vi "test TCX read (installed 71).vi"() -> ()   [LabVIEW 2011] (continued)
><Trackpoint><Time>2008-03-03T14:08:26Z</Time><Position><LatitudeDegrees>35.866312</LatitudeDegrees><LongitudeDegrees>-78.880611</LongitudeDegrees></Position><AltitudeMeters>99.153</AltitudeMeters><DistanceMeters>10693.477</DistanceMeters><Cadence>84</Cadence><Extensions><TPX xmlns=\"http://www.garmin.com/xmlschemas/ActivityExtension/v2\"><Watts>141</Watts></TPX></Extensions></Trackpoint><Trackpoint><Time>2008-03-03T14:08:27Z</Time><Position><LatitudeDegrees>35.866343</LatitudeDegrees><LongitudeDegrees>-78.880503</LongitudeDegrees></Position><AltitudeMeters>99.153</AltitudeMeters><DistanceMeters>10703.830</DistanceMeters><Cadence>84</Cadence><Extensions><TPX xmlns=\"http://www.garmin.com/xmlschemas/ActivityExtension/v2\"><Watts>141</Watts></TPX></Extensions></Trackpoint><Trackpoint><Time>2008-03-03T14:08:28Z</Time><Position><LatitudeDegrees>35.866345</LatitudeDegrees><LongitudeDegrees>-78.880391</LongitudeDegrees></Position><AltitudeMeters>99.153</AltitudeMeters><DistanceMeters>10713.883</DistanceMeters><Cadence>38</Cadence><Extensions><TPX xmlns=\"http://www.garmin.com/xmlschemas/ActivityExtension/v2\"><Watts>13</Watts></TPX></Extensions></Trackpoint><Trackpoint><Time>2008-03-03T14:08:29Z</Time><Position><LatitudeDegrees>35.866328</LatitudeDegrees><LongitudeDegrees>-78.880294</LongitudeDegrees></Position><AltitudeMeters>99.634</AltitudeMeters><DistanceMeters>10722.747</DistanceMeters><Cadence>36</Cadence><Extensions><TPX xmlns=\"http://www.garmin.com/xmlschemas/ActivityExtension/v2\"><Watts>26</Watts></TPX></Extensions></Trackpoint><Trackpoint><Time>2008-03-03T14:08:30Z</Time><Position><LatitudeDegrees>35.866278</LatitudeDegrees><LongitudeDegrees>-78.880221</LongitudeDegrees></Position><AltitudeMeters>99.634</AltitudeMeters><DistanceMeters>10730.963</DistanceMeters><Cadence>36</Cadence><Extensions><TPX xmlns=\"http://www.garmin.com/xmlschemas/ActivityExtension/v2\"><Watts>25</Watts></TPX></Extensions></Trackpoint><Trackpoint><Time>2008-03-03T14:08:31Z</Time><Position><LatitudeDegrees>35.866190</LatitudeDegrees><LongitudeDegrees>-78.880183</LongitudeDegrees></Position><AltitudeMeters>99.634</AltitudeMeters><DistanceMeters>10741.313</DistanceMeters><Cadence>74</Cadence><Extensions><TPX xmlns=\"http://www.garmin.com/xmlschemas/ActivityExtension/v2\"><Watts>115</Watts></TPX></Extensions></Trackpoint><Trackpoint><Time>2008-03-03T14:08:32Z</Time><Position><LatitudeDegrees>35.866105</LatitudeDegrees><LongitudeDegrees>-78.880147</LongitudeDegrees></Position><AltitudeMeters>99.634</AltitudeMeters><DistanceMeters>10751.273</DistanceMeters><Cadence>74</Cadence><Extensions><TPX xmlns=\"http://www.garmin.com/xmlschemas/ActivityExtension/v2\"><Watts>166</Watts></TPX></Extensions></Trackpoint><Trackpoint><Time>2008-03-03T14:08:33Z</Time><Position><LatitudeDegrees>35.866021</LatitudeDegrees><LongitudeDegrees>-78.880110</LongitudeDegrees></Position><AltitudeMeters>100.115</AltitudeMeters><DistanceMeters>10761.154</DistanceMeters><Cadence>75</Cadence><Extensions><TPX xmlns=\"http://www.garmin.com/xmlschemas/ActivityExtension/v2\"><Watts>323</Watts></TPX></Extensions></Trackpoint><Trackpoint><Time>2008-03-03T14:08:34Z</Time><Position><LatitudeDegrees>35.865940</LatitudeDegrees><LongitudeDegrees>-78.880073</LongitudeDegrees></Position><AltitudeMeters>99.634</AltitudeMeters><DistanceMeters>10770.754</DistanceMeters><Cadence>76</Cadence><Extensions><TPX xmlns=\"http://www.garmin.com/xmlschemas/ActivityExtension/v2\"><Watts>355</Watts></TPX></Extensions></Trackpoint><Trackpoint><Time>2008-03-03T14:08:35Z</Time><Position><LatitudeDegrees>35.865853</LatitudeDegrees><LongitudeDegrees>-78.880034</LongitudeDegrees></Position><AltitudeMeters>100.115</AltitudeMeters><DistanceMeters>10781.071</DistanceMeters><Cadence>77</Cadence><Extensions><TPX xmlns=\"http://www.garmin.com/xmlschemas/ActivityExtension/v2\"><Watts>333</Watts></TPX></Extensions></Trackpoint><Trackpoint><Time>2008-03-03T14:08:36Z</Time><Position><LatitudeDegrees>35.865737</LatitudeDegrees><LongitudeDegrees>-78.879989</LongitudeDegrees></Position><AltitudeMeters>99.153</AltitudeMeters><DistanceMeters>10794.555</DistanceMeters><Cadence>80</Cadence><Extensions><TPX xmlns=\"http://www.garmin.com/xmlschemas/ActivityExtension/v2\"><Watts>223</Watts></TPX></Extensions></Trackpoint><Trackpoint><Time>2008-03-03T14:08:37Z</Time><Position><LatitudeDegrees>35.865638</LatitudeDegrees><LongitudeDegrees>-78.879966</LongitudeDegrees></Position><AltitudeMeters>99.634</AltitudeMeters><DistanceMeters>10805.750</DistanceMeters><Cadence>80</Cadence><Extensions><TPX xmlns=\"http://www.garmin.com/xmlschemas/ActivityExtension/v2\"><Watts>223</Watts></TPX></Extensions></Trackpoint><Trackpoint><Time>2008-03-03T14:08:38Z</Time><Position><LatitudeDegrees>35.865555</LatitudeDegrees><LongitudeDegrees>-78.879967</LongitudeDegrees></Position><AltitudeMeters>98.672</AltitudeMeters><DistanceMeters>10814.789</DistanceMeters><Cadence>83</Cadence><Extensions><TPX xmlns=\"http://www.garmin.com/xmlschemas/ActivityExtension/v2\"><Watts>157</Watts></TPX></Extensions></Trackpoint><Trackpoint><Time>2008-03-03T14:08:39Z</Time><Position><LatitudeDegrees>35.865453</LatitudeDegrees><LongitudeDegrees>-78.879945</LongitudeDegrees></Position><AltitudeMeters>98.672</AltitudeMeters><DistanceMeters>10826.345</DistanceMeters><Cadence>80</Cadence><Extensions><TPX xmlns=\"http://www.garmin.com/xmlschemas/ActivityExtension/v2\"><Watts>148</Watts></TPX></Extensions></Trackpoint><Trackpoint><Time>2008-03-03T14:08:40Z</Time><Position><LatitudeDegrees>35.865353</LatitudeDegrees><LongitudeDegrees>-78.879923</LongitudeDegrees></Position><AltitudeMeters>98.192</AltitudeMeters><DistanceMeters>10837.629</DistanceMeters><Cadence>80</Cadence><Extensions><TPX xmlns=\"http://www.garmin.com/xmlschemas/ActivityExtension/v2\"><Watts>147</Watts></TPX></Extensions></Trackpoint><Trackpoint><Time>2008-03-03T14:08:41Z</Time><Position><LatitudeDegrees>35.865256</LatitudeDegrees><LongitudeDegrees>-78.879904</LongitudeDegrees></Position><AltitudeMeters>97.711</AltitudeMeters><DistanceMeters>10848.521</DistanceMeters><Cadence>85</Cadence><Extensions><TPX xmlns=\"http://www.garmin.com/xmlschemas/ActivityExtension/v2\"><Watts>133</Watts></TPX></Extensions></Trackpoint><Trackpoint><Time>2008-03-03T14:08:42Z</Time><Position><LatitudeDegrees>35.865159</LatitudeDegrees><LongitudeDegrees>-78.879884</LongitudeDegrees></Position><AltitudeMeters>96.750</AltitudeMeters><DistanceMeters>10859.452</DistanceMeters><Cadence>86</Cadence><Extensions><TPX xmlns=\"http://www.garmin.com/xmlschemas/ActivityExtension/v2\"><Watts>132</Watts></TPX></Extensions></Trackpoint><Trackpoint><Time>2008-03-03T14:08:43Z</Time><Position><LatitudeDegrees>35.865057</LatitudeDegrees><LongitudeDegrees>-78.879859</LongitudeDegrees></Position><AltitudeMeters>96.269</AltitudeMeters><DistanceMeters>10871.032</DistanceMeters><Cadence>88</Cadence><Extensions><TPX xmlns=\"http://www.garmin.com/xmlschemas/ActivityExtension/v2\"><Watts>100</Watts></TPX></Extensions></Trackpoint><Trackpoint><Time>2008-03-03T14:08:44Z</Time><Position><LatitudeDegrees>35.864950</LatitudeDegrees><LongitudeDegrees>-78.879828</LongitudeDegrees></Position><AltitudeMeters>95.788</AltitudeMeters><DistanceMeters>10883.138</DistanceMeters><Cadence>84</Cadence><Extensions><TPX xmlns=\"http://www.garmin.com/xmlschemas/ActivityExtension/v2\"><Watts>105</Watts></TPX></Extensions></Trackpoint><Trackpoint><Time>2008-03-03T14:08:45Z</Time><Position><LatitudeDegrees>35.864843</LatitudeDegrees><LongitudeDegrees>-78.879794</LongitudeDegrees></Position><AltitudeMeters>96.269</AltitudeMeters><DistanceMeters>10895.494</DistanceMeters><Cadence>86</Cadence><Extensions><TPX xmlns=\"http://www.garmin.com/xmlschemas/ActivityExtension/v2\"><Watts>123</Watts></TPX></Extensions></Trackpoint><Trackpoint><Time>2008-03-03T14:08:46Z</Time><Position><LatitudeDegrees>35.864733</LatitudeDegrees><LongitudeDegrees>-78.879755</LongitudeDegrees></Position><AltitudeMeters>95.308</AltitudeMeters><DistanceMeters>10908.254</DistanceMeters><Cadence>88</Cadence><Extensions><TPX xmlns=\"http://www.garmin.com/xmlschemas/ActivityExtension/v2\"><Watts>150</Watts></TPX></Extensions></Trackpoint><Trackpoint><Time>2008-03-03T14:08:47Z</Time><Position><LatitudeDegrees>35.864616</LatitudeDegrees><LongitudeDegrees>-78.879705</LongitudeDegrees></Position><AltitudeMeters>94.827</AltitudeMeters><DistanceMeters>10921.946</DistanceMeters><Cadence>88</Cadence><Extensions><TPX xmlns=\"http://www.garmin.com/xmlschemas/ActivityExtension/v2\"><Watts>151</Watts></TPX></Extensions></Trackpoint><Trackpoint><Time>2008-03-03T14:08:48Z</Time><Position><LatitudeDegrees>35.864512</LatitudeDegrees><LongitudeDegrees>-78.879645</LongitudeDegrees></Position><AltitudeMeters>94.347</AltitudeMeters><DistanceMeters>10934.686</DistanceMeters><Cadence>91</Cadence><Extensions><TPX xmlns=\"http://www.garmin.com/xmlschemas/ActivityExtension/v2\"><Watts>156</Watts></TPX></Extensions></Trackpoint><Trackpoint><Time>2008-03-03T14:08:49Z</Time><Position><LatitudeDegrees>35.864420</LatitudeDegrees><LongitudeDegrees>-78.879574</LongitudeDegrees></Position><AltitudeMeters>94.347</AltitudeMeters><DistanceMeters>10946.729</DistanceMeters><Cadence>91</Cadence><Extensions><TPX xmlns=\"http://www.garmin.com/xmlschemas/ActivityExtension/v2\"><Watts>158</Watts></TPX></Extensions></Trackpoint><Trackpoint><Time>2008-03-03T14:08:50Z</Time><Position><LatitudeDegrees>35.864328</LatitudeDegrees><LongitudeDegrees>-78.879493</LongitudeDegrees></Position><AltitudeMeters>94.347</AltitudeMeters><DistanceMeters>10959.344</DistanceMeters><Cadence>91</Cadence><Extensions><TPX xmlns=\"http://www.garmin.com/xmlschemas/ActivityExtension/v2\"><Watts>129</Watts></TPX></Extensions></Trackpoint><Trackpoint><Time>2008-03-03T14:08:51Z</Time><Position><LatitudeDegrees>35.864240</LatitudeDegrees><LongitudeDegrees>-78.879401</LongitudeDegrees></Position><AltitudeMeters>93.385</AltitudeMeters><DistanceMeters>10972.160</DistanceMeters><Cadence>90</Cadence><Extensions><TPX xmlns=\"http://www.garmin.com/xmlschemas/ActivityExtension/v2\"><Watts>124</Watts></TPX></Extensions></Trackpoint><Trackpoint><Time>2008-03-03T14:08:52Z</Time><Position><LatitudeDegrees>35.864158</LatitudeDegrees><LongitudeDegrees>-78.879305</LongitudeDegrees></Position><AltitudeMeters>92.424</AltitudeMeters><DistanceMeters>10984.663</DistanceMeters><Cadence>90</Cadence><Extensions><TPX xmlns=\"http://www.garmin.com/xmlschemas/ActivityExtension/v2\"><Watts>123</Watts></TPX></Extensions></Trackpoint><Trackpoint><Time>2008-03-03T14:08:53Z</Time><Position><LatitudeDegrees>35.864078</LatitudeDegrees><LongitudeDegrees>-78.879213</LongitudeDegrees></Position><AltitudeMeters>92.424</AltitudeMeters><DistanceMeters>10996.836</DistanceMeters><Cadence>87</Cadence><Extensions><TPX xmlns=\"http://www.garmin.com/xmlschemas/ActivityExtension/v2\"><Watts>124</Watts></TPX></Extensions></Trackpoint><Trackpoint><Time>2008-03-03T14:08:54Z</Time><Position><LatitudeDegrees>35.863996</LatitudeDegrees><LongitudeDegrees>-78.879127</LongitudeDegrees></Position><AltitudeMeters>92.424</AltitudeMeters><DistanceMeters>11008.705</DistanceMeters><Cadence>87</Cadence><Extensions><TPX xmlns=\"http://www.garmin.com/xmlschemas/ActivityExtension/v2\"><Watts>124</Watts></TPX></Extensions></Trackpoint><Trackpoint><Time>2008-03-03T14:08:55Z</Time><Position><LatitudeDegrees>35.863928</LatitudeDegrees><LongitudeDegrees>-78.879033</LongitudeDegrees></Position><AltitudeMeters>92.424</AltitudeMeters><DistanceMeters>11020.062</DistanceMeters><Cadence>0</Cadence></Trackpoint><Trackpoint><Time>2008-03-03T14:08:56Z</Time><Position><LatitudeDegrees>35.863913</LatitudeDegrees><LongitudeDegrees>-78.878926</LongitudeDegrees></Position><AltitudeMeters>91.463</AltitudeMeters><DistanceMeters>11029.886</DistanceMeters><Cadence>0</Cadence></Trackpoint><Trackpoint><Time>2008-03-03T14:08:57Z</Time><Position><LatitudeDegrees>35.863940</LatitudeDegrees><LongitudeDegrees>-78.878817</LongitudeDegrees></Position><AltitudeMeters>90.982</AltitudeMeters><DistanceMeters>11040.122</DistanceMeters><Cadence>14</Cadence><Extensions><TPX xmlns=\"http://www.garmin.com/xmlschemas/ActivityExtension/v2\"><Watts>4</Watts></TPX></Extensions></Trackpoint><Trackpoint><Time>2008-03-03T14:08:58Z</Time><Position><LatitudeDegrees>35.864012</LatitudeDegrees><LongitudeDegrees>-78.878736</LongitudeDegrees></Position><AltitudeMeters>90.982</AltitudeMeters><DistanceMeters>11051.058</DistanceMeters><Cadence>73</Cadence><Extensions><TPX xmlns=\"http://www.garmin.com/xmlschemas/ActivityExtension/v2\"><Watts>88</Watts></TPX></Extensions></Trackpoint><Trackpoint><Time>2008-03-03T14:08:59Z</Time><Position><LatitudeDegrees>35.864082</LatitudeDegrees><LongitudeDegrees>-78.878660</LongitudeDegrees></Position><AltitudeMeters>90.982</AltitudeMeters><DistanceMeters>11061.331</DistanceMeters><Cadence>74</Cadence><Extensions><TPX xmlns=\"http://www.garmin.com/xmlschemas/ActivityExtension/v2\"><Watts>121</Watts></TPX></Extensions></Trackpoint><Trackpoint><Time>2008-03-03T14:09:00Z</Time><Position><LatitudeDegrees>35.864150</LatitudeDegrees><LongitudeDegrees>-78.878573</LongitudeDegrees></Position><AltitudeMeters>90.982</AltitudeMeters><DistanceMeters>11072.221</DistanceMeters><Cadence>75</Cadence><Extensions><TPX xmlns=\"http://www.garmin.com/xmlschemas/ActivityExtension/v2\"><Watts>284</Watts></TPX></Extensions></Trackpoint><Trackpoint><Time>2008-03-03T14:09:01Z</Time><Position><LatitudeDegrees>35.864204</LatitudeDegrees><LongitudeDegrees>-78.878489</LongitudeDegrees></Position><AltitudeMeters>91.463</AltitudeMeters><DistanceMeters>11081.919</DistanceMeters><Cadence>76</Cadence><Extensions><TPX xmlns=\"http://www.garmin.com/xmlschemas/ActivityExtension/v2\"><Watts>444</Watts></TPX></Extensions></Trackpoint><Trackpoint><Time>2008-03-03T14:09:02Z</Time><Position><LatitudeDegrees>35.864256</LatitudeDegrees><LongitudeDegrees>-78.878400</LongitudeDegrees></Position><AltitudeMeters>91.943</AltitudeMeters><DistanceMeters>11091.741</DistanceMeters><Cadence>78</Cadence><Extensions><TPX xmlns=\"http://www.garmin.com/xmlschemas/ActivityExtension/v2\"><Watts>540</Watts></TPX></Extensions></Trackpoint><Trackpoint><Time>2008-03-03T14:09:03Z</Time><Position><LatitudeDegrees>35.864308</LatitudeDegrees><LongitudeDegrees>-78.878311</LongitudeDegrees></Position><AltitudeMeters>91.463</AltitudeMeters><DistanceMeters>11101.723</DistanceMeters><Cadence>79</Cadence><Extensions><TPX xmlns=\"http://www.garmin.com/xmlschemas/ActivityExtension/v2\"><Watts>529</Watts></TPX></Extensions></Trackpoint><Trackpoint><Time>2008-03-03T14:09:04Z</Time><Position><LatitudeDegrees>35.864360</LatitudeDegrees><LongitudeDegrees>-78.878217</LongitudeDegrees></Position><AltitudeMeters>91.943</AltitudeMeters><DistanceMeters>11111.980</DistanceMeters><Cadence>79</Cadence><Extensions><TPX xmlns=\"http://www.garmin.com/xmlschemas/ActivityExtension/v2\"><Watts>526</Watts></TPX></Extensions></Trackpoint><Trackpoint><Time>2008-03-03T14:09:05Z</Time><Position><LatitudeDegrees>35.864407</LatitudeDegrees><LongitudeDegrees>-78.878122</LongitudeDegrees></Position><AltitudeMeters>91.943</AltitudeMeters><DistanceMeters>11121.941</DistanceMeters><Cadence>79</Cadence><Extensions><TPX xmlns=\"http://www.garmin.com/xmlschemas/ActivityExtension/v2\"><Watts>475</Watts></TPX></Extensions></Trackpoint><Trackpoint><Time>2008-03-03T14:09:06Z</Time><Position><LatitudeDegrees>35.864447</LatitudeDegrees><LongitudeDegrees>-78.878027</LongitudeDegrees></Position><AltitudeMeters>92.424</AltitudeMeters><DistanceMeters>11131.617</DistanceMeters><Cadence>80</Cadence><Extensions><TPX xmlns=\"http://www.garmin.com/xmlschemas/ActivityExtension/v2\"><Watts>446</Watts></TPX></Extensions></Trackpoint><Trackpoint><Time>2008-03-03T14:09:07Z</Time><Position><LatitudeDegrees>35.864487</LatitudeDegrees><LongitudeDegrees>-78.877926</LongitudeDegrees></Position><AltitudeMeters>92.424</AltitudeMeters><DistanceMeters>11141.777</DistanceMeters><Cadence>80</Cadence><Extensions><TPX xmlns=\"http://www.garmin.com/xmlschemas/ActivityExtension/v2\"><Watts>438</Watts></TPX></Extensions></Trackpoint><Trackpoint><Time>2008-03-03T14:09:08Z</Time><Position><LatitudeDegrees>35.864523</LatitudeDegrees><LongitudeDegrees>-78.877825</LongitudeDegrees></Position><AltitudeMeters>92.424</AltitudeMeters><DistanceMeters>11151.760</DistanceMeters><Cadence>82</Cadence><Extensions><TPX xmlns=\"http://www.garmin.com/xmlschemas/ActivityExtension/v2\"><Watts>413</Watts></TPX></Extensions></Trackpoint><Trackpoint><Time>2008-03-03T14:09:09Z</Time><Position><LatitudeDegrees>35.864554</LatitudeDegrees><LongitudeDegrees>-78.877724</LongitudeDegrees></Position><AltitudeMeters>92.424</AltitudeMeters><DistanceMeters>11161.466</DistanceMeters><Cadence>80</Cadence><Extensions><TPX xmlns=\"http://www.garmin.com/xmlschemas/ActivityExtension/v2\"><Watts>336</Watts></TPX></Extensions></Trackpoint><Trackpoint><Time>2008-03-03T14:09:10Z</Time><Position><LatitudeDegrees>35.864575</LatitudeDegrees><LongitudeDegrees>-78.877624</LongitudeDegrees></Position><AltitudeMeters>91.943</AltitudeMeters><DistanceMeters>11170.762</DistanceMeters><Cadence>80</Cadence><Extensions><TPX xmlns=\"http://www.garmin.com/xmlschemas/ActivityExtension/v2\"><Watts>333</Watts></TPX></Extensions></Trackpoint><Trackpoint><Time>2008-03-03T14:09:11Z</Time><Position><LatitudeDegrees>35.864602</LatitudeDegrees><LongitudeDegrees>-78.877526</LongitudeDegrees></Position><AltitudeMeters>91.943</AltitudeMeters><DistanceMeters>11180.042</DistanceMeters><Cadence>0</Cadence></Trackpoint><Trackpoint><Time>2008-03-03T14:09:12Z</Time><Position><LatitudeDegrees>35.864627</LatitudeDegrees><LongitudeDegrees>-78.877434</LongitudeDegrees></Position><AltitudeMeters>91.463</AltitudeMeters><DistanceMeters>11188.773</DistanceMeters><Cadence>0</Cadence></Trackpoint><Trackpoint><Time>2008-03-03T14:09:13Z</Time><Position><LatitudeDegrees>35.864647</LatitudeDegrees><LongitudeDegrees>-78.877351</LongitudeDegrees></Position><AltitudeMeters>91.463</AltitudeMeters><DistanceMeters>11196.600</DistanceMeters><Cadence>0</Cadence></Trackpoint><Trackpoint><Time>2008-03-03T14:09:14Z</Time><Position><LatitudeDegrees>35.864661</LatitudeDegrees><LongitudeDegrees>-78.877279</LongitudeDegrees></Position><AltitudeMeters>90.982</AltitudeMeters><DistanceMeters>11203.146</DistanceMeters><Cadence>0</Cadence></Trackpoint><Trackpoint><Time>2008-03-03T14:09:15Z</Time><Position><LatitudeDegrees>35.864669</LatitudeDegrees><LongitudeDegrees>-78.877219</LongitudeDegrees></Position><AltitudeMeters>90.982</AltitudeMeters><DistanceMeters>11208.569</DistanceMeters><Cadence>0</Cadence></Trackpoint><Trackpoint><Time>2008-03-03T14:09:16Z</Time><Position><LatitudeDegrees>35.864665</LatitudeDegrees><LongitudeDegrees>-78.877171</LongitudeDegrees></Position><AltitudeMeters>90.501</AltitudeMeters><DistanceMeters>11212.869</DistanceMeters><Cadence>0</Cadence></Trackpoint><Trackpoint><Time>2008-03-03T14:09:17Z</Time><Position><LatitudeDegrees>35.864650</LatitudeDegrees><LongitudeDegrees>-78.877146</LongitudeDegrees></Position><AltitudeMeters>90.501</AltitudeMeters><DistanceMeters>11215.633</DistanceMeters><Cadence>0</Cadence></Trackpoint><Trackpoint><Time>2008-03-03T14:09:18Z</Time><Position><LatitudeDegrees>35.864641</LatitudeDegrees><LongitudeDegrees>-78.877137</LongitudeDegrees></Position><AltitudeMeters>90.501</AltitudeMeters><DistanceMeters>11216.748</DistanceMeters><Cadence>0</Cadence></Trackpoint><Trackpoint><Time>2008-03-03T14:09:19Z</Time><Position><LatitudeDegrees>35.864638</LatitudeDegrees><LongitudeDegrees>-78.877137</LongitudeDegrees></Position><AltitudeMeters>90.501</AltitudeMeters><DistanceMeters>11216.885</DistanceMeters><Cadence>0</Cadence></Trackpoint><Trackpoint><Time>2008-03-03T14:09:20Z</Time><Position><LatitudeDegrees>35.864636</LatitudeDegrees><LongitudeDegrees>-78.877141</LongitudeDegrees></Position><AltitudeMeters>90.021</AltitudeMeters><DistanceMeters>11217.296</DistanceMeters></Trackpoint><Trackpoint><Time>2008-03-03T14:09:21Z</Time><Position><LatitudeDegrees>35.864632</LatitudeDegrees><LongitudeDegrees>-78.877145</LongitudeDegrees></Position><AltitudeMeters>90.501</AltitudeMeters><DistanceMeters>11217.786</DistanceMeters></Trackpoint><Trackpoint><Time>2008-03-03T14:09:22Z</Time></Trackpoint><Trackpoint><Time>2008-03-03T14:09:23Z</Time><Position><LatitudeDegrees>35.864631</LatitudeDegrees><LongitudeDegrees>-78.877146</LongitudeDegrees></Position><AltitudeMeters>90.021</AltitudeMeters><DistanceMeters>11217.786</DistanceMeters></Trackpoint><Trackpoint><Time>2008-03-03T23:05:22Z</Time></Trackpoint><Trackpoint><Time>2008-03-03T23:05:23Z</Time><Position><LatitudeDegrees>35.864599</LatitudeDegrees><LongitudeDegrees>-78.877183</LongitudeDegrees></Position><AltitudeMeters>88.579</AltitudeMeters><DistanceMeters>11217.786</DistanceMeters></Trackpoint></Track></Lap><Lap StartTime=\"2008-03-03T23:05:23Z\"><TotalTimeSeconds>1256.30</TotalTimeSeconds><DistanceMeters>11205.165039</DistanceMeters><MaximumSpeed>14.865000</MaximumSpeed><Calories>380</Calories><Intensity>Active</Intensity><Cadence>76</Cadence><TriggerMethod>Manual</TriggerMethod><Track><Trackpoint><Time>2008-03-03T23:05:24Z</Time><Position><LatitudeDegrees>35.864599</LatitudeDegrees><LongitudeDegrees>-78.877182</LongitudeDegrees></Position><AltitudeMeters>65.026</AltitudeMeters><DistanceMeters>11217.828</DistanceMeters></Trackpoint><Trackpoint><Time>2008-03-03T23:05:25Z</Time><Position><LatitudeDegrees>35.864599</LatitudeDegrees><LongitudeDegrees>-78.877182</LongitudeDegrees></Position><AltitudeMeters>65.026</AltitudeMeters><DistanceMeters>11217.846</DistanceMeters></Trackpoint><Trackpoint><Time>2008-03-03T23:05:26Z</Time><Position><LatitudeDegrees>35.864599</LatitudeDegrees><LongitudeDegrees>-78.877181</LongitudeDegrees></Position><AltitudeMeters>65.026</AltitudeMeters><DistanceMeters>11217.897</DistanceMeters></Trackpoint><Trackpoint><Time>2008-03-03T23:05:27Z</Time><Position><LatitudeDegrees>35.864600</LatitudeDegrees><LongitudeDegrees>-78.877183</LongitudeDegrees></Position><AltitudeMeters>65.026</AltitudeMeters><DistanceMeters>11218.080</DistanceMeters></Trackpoint><Trackpoint><Time>2008-03-03T23:05:28Z</Time><Position><LatitudeDegrees>35.864598</LatitudeDegrees><LongitudeDegrees>-78.877196</LongitudeDegrees></Position><AltitudeMeters>65.026</AltitudeMeters><DistanceMeters>11219.385</DistanceMeters></Trackpoint><Trackpoint><Time>2008-03-03T23:05:29Z</Time><Position><LatitudeDegrees>35.864596</LatitudeDegrees><LongitudeDegrees>-78.877215</LongitudeDegrees></Position><AltitudeMeters>65.026</AltitudeMeters><DistanceMeters>11221.062</DistanceMeters></Trackpoint><Trackpoint><Time>2008-03-03T23:05:30Z</Time><Position><LatitudeDegrees>35.864600</LatitudeDegrees><LongitudeDegrees>-78.877227</LongitudeDegrees></Position><AltitudeMeters>65.026</AltitudeMeters><DistanceMeters>11222.095</DistanceMeters></Trackpoint><Trackpoint><Time>2008-03-03T23:05:31Z</Time><Position><LatitudeDegrees>35.864611</LatitudeDegrees><LongitudeDegrees>-78.877234</LongitudeDegrees></Position><AltitudeMeters>65.026</AltitudeMeters><DistanceMeters>11223.448</DistanceMeters><Cadence>2</Cadence><Extensions><TPX xmlns=\"http://www.garmin.com/xmlschemas/ActivityExtension/v2\"><Watts>194</Watts></TPX></Extensions></Trackpoint><Trackpoint><Time>2008-03-03T23:05:32Z</Time><Position><LatitudeDegrees>35.864624</LatitudeDegrees><LongitudeDegrees>-78.877245</LongitudeDegrees></Position><AltitudeMeters>65.026</AltitudeMeters><DistanceMeters>11225.238</DistanceMeters><Cadence>2</Cadence><Extensions><TPX xmlns=\"http://www.garmin.com/xmlschemas/ActivityExtension/v2\"><Watts>193</Watts></TPX></Extensions></Trackpoint><Trackpoint><Time>2008-03-03T23:05:33Z</Time><Position><LatitudeDegrees>35.864635</LatitudeDegrees><LongitudeDegrees>-78.877267</LongitudeDegrees></Position><AltitudeMeters>65.507</AltitudeMeters><DistanceMeters>11227.559</DistanceMeters><Cadence>0</Cadence></Trackpoint><Trackpoint><Time>2008-03-03T23:05:34Z</Time><Position><LatitudeDegrees>35.864638</LatitudeDegrees><LongitudeDegrees>-78.877295</LongitudeDegrees></Position><AltitudeMeters>65.507</AltitudeMeters><DistanceMeters>11230.062</DistanceMeters><Cadence>20</Cadence><Extensions><TPX xmlns=\"http://www.garmin.com/xmlschemas/ActivityExtension/v2\"><Watts>103</Watts></TPX></Extensions></Trackpoint><Trackpoint><Time>2008-03-03T23:05:35Z</Time><Position><LatitudeDegrees>35.864634</LatitudeDegrees><LongitudeDegrees>-78.877330</LongitudeDegrees></Position><AltitudeMeters>65.507</AltitudeMeters><DistanceMeters>11233.309</DistanceMeters><Cadence>44</Cadence><Extensions><TPX xmlns=\"http://www.garmin.com/xmlschemas/ActivityExtension/v2\"><Watts>320</Watts></TPX></Extensions></Trackpoint><Trackpoint><Time>2008-03-03T23:05:36Z</Time><Position><LatitudeDegrees>35.864623</LatitudeDegrees><LongitudeDegrees>-78.877377</LongitudeDegrees></Position><AltitudeMeters>65.507</AltitudeMeters><DistanceMeters>11237.704</DistanceMeters><Cadence>60</Cadence><Extensions><TPX xmlns=\"http://www.garmin.com/xmlschemas/ActivityExtension/v2\"><Watts>420</Watts></TPX></Extensions></Trackpoint><Trackpoint><Time>2008-03-03T23:05:37Z</Time><Position><LatitudeDegrees>35.864609</LatitudeDegrees><LongitudeDegrees>-78.877434</LongitudeDegrees></Position><AltitudeMeters>65.988</AltitudeMeters><DistanceMeters>11243.220</DistanceMeters><Cadence>60</Cadence><Extensions><TPX xmlns=\"http://www.garmin.com/xmlschemas/ActivityExtension/v2\"><Watts>416</Watts></TPX></Extensions></Trackpoint><Trackpoint><Time>2008-03-03T23:05:38Z</Time><Position><LatitudeDegrees>35.864592</LatitudeDegrees><LongitudeDegrees>-78.877503</LongitudeDegrees></Position><AltitudeMeters>65.988</AltitudeMeters><DistanceMeters>11249.730</DistanceMeters><Cadence>81</Cadence><Extensions><TPX xmlns=\"http://www.garmin.com/xmlschemas/ActivityExtension/v2\"><Watts>637</Watts></TPX></Extensions></Trackpoint><Trackpoint><Time>2008-03-03T23:05:39Z</Time><Position><LatitudeDegrees>35.864574</LatitudeDegrees><LongitudeDegrees>-78.877580</LongitudeDegrees></Position><AltitudeMeters>66.468</AltitudeMeters><DistanceMeters>11257.070</DistanceMeters><Cadence>85</Cadence><Extensions><TPX xmlns=\"http://www.garmin.com/xmlschemas/ActivityExtension/v2\"><Watts>651</Watts></TPX></Extensions></Trackpoint><Trackpoint><Time>2008-03-03T23:05:40Z</Time><Position><LatitudeDegrees>35.864553</LatitudeDegrees><LongitudeDegrees>-78.877662</LongitudeDegrees></Position><AltitudeMeters>66.949</AltitudeMeters><DistanceMeters>11264.834</DistanceMeters><Cadence>72</Cadence><Extensions><TPX xmlns=\"http://www.garmin.com/xmlschemas/ActivityExtension/v2\"><Watts>566</Watts></TPX></Extensions></Trackpoint><Trackpoint><Time>2008-03-03T23:05:41Z</Time><Position><LatitudeDegrees>35.864529</LatitudeDegrees><LongitudeDegrees>-78.877747</LongitudeDegrees></Position><AltitudeMeters>66.949</AltitudeMeters><DistanceMeters>11272.925</DistanceMeters><Cadence>75</Cadence><Extensions><TPX xmlns=\"http://www.garmin.com/xmlschemas/ActivityExtension/v2\"><Watts>522</Watts></TPX></Extensions></Trackpoint><Trackpoint><Time>2008-03-03T23:05:42Z</Time><Position><LatitudeDegrees>35.864500</LatitudeDegrees><LongitudeDegrees>-78.877836</LongitudeDegrees></Position><AltitudeMeters>66.949</AltitudeMeters><DistanceMeters>11281.620</DistanceMeters><Cadence>80</Cadence><Extensions><TPX xmlns=\"http://www.garmin.com/xmlschemas/ActivityExtension/v2\"><Watts>518</Watts></TPX></Extensions></Trackpoint><Trackpoint><Time>2008-03-03T23:05:43Z</Time><Position><LatitudeDegrees>35.864469</LatitudeDegrees><LongitudeDegrees>-78.877929</LongitudeDegrees></Position><AltitudeMeters>66.949</AltitudeMeters><DistanceMeters>11290.788</DistanceMeters><Cadence>86</Cadence><Extensions><TPX xmlns=\"http://www.garmin.com/xmlschemas/ActivityExtension/v2\"><Watts>564</Watts></TPX></Extensions></Trackpoint><Trackpoint><Time>2008-03-03T23:05:44Z</Time><Position><LatitudeDegrees>35.864435</LatitudeDegrees><LongitudeDegrees>-78.878027</LongitudeDegrees></Position><AltitudeMeters>66.949</AltitudeMeters><DistanceMeters>11300.357</DistanceMeters><Cadence>88</Cadence><Extensions><TPX xmlns=\"http://www.garmin.com/xmlschemas/ActivityExtension/v2\"><Watts>556</Watts></TPX></Extensions></Trackpoint><Trackpoint><Time>2008-03-03T23:05:45Z</Time><Position><LatitudeDegrees>35.864399</LatitudeDegrees><LongitudeDegrees>-78.878127</LongitudeDegrees></Position><AltitudeMeters>67.430</AltitudeMeters><DistanceMeters>11310.256</DistanceMeters><Cadence>91</Cadence><Extensions><TPX xmlns=\"http://www.garmin.com/xmlschemas/ActivityExtension/v2\"><Watts>521</Watts></TPX></Extensions></Trackpoint><Trackpoint><Time>2008-03-03T23:05:46Z</Time><Position><LatitudeDegrees>35.864360</LatitudeDegrees><LongitudeDegrees>-78.878227</LongitudeDegrees></Position><AltitudeMeters>67.430</AltitudeMeters><DistanceMeters>11320.329</DistanceMeters><Cadence>86</Cadence><Extensions><TPX xmlns=\"http://www.garmin.com/xmlschemas/ActivityExtension/v2\"><Watts>484</Watts></TPX></Extensions></Trackpoint><Trackpoint><Time>2008-03-03T23:05:47Z</Time><Position><LatitudeDegrees>35.864317</LatitudeDegrees><LongitudeDegrees>-78.878326</LongitudeDegrees></Position><AltitudeMeters>67.430</AltitudeMeters><DistanceMeters>11330.483</DistanceMeters><Cadence>86</Cadence><Extensions><TPX xmlns=\"http://www.garmin.com/xmlschemas/ActivityExtension/v2\"><Watts>487</Watts></TPX></Extensions></Trackpoint><Trackpoint><Time>2008-03-03T23:05:48Z</Time><Position><LatitudeDegrees>35.864267</LatitudeDegrees><LongitudeDegrees>-78.878422</LongitudeDegrees></Position><AltitudeMeters>66.949</AltitudeMeters><DistanceMeters>11340.710</DistanceMeters><Cadence>83</Cadence><Extensions><TPX xmlns=\"http://www.garmin.com/xmlschemas/ActivityExtension/v2\"><Watts>282</Watts></TPX></Extensions></Trackpoint><Trackpoint><Time>2008-03-03T23:05:49Z</Time><Position><LatitudeDegrees>35.864211</LatitudeDegrees><LongitudeDegrees>-78.878514</LongitudeDegrees></Position><AltitudeMeters>66.949</AltitudeMeters><DistanceMeters>11351.038</DistanceMeters><Cadence>84</Cadence><Extensions><TPX xmlns=\"http://www.garmin.com/xmlschemas/ActivityExtension/v2\"><Watts>235</Watts></TPX></Extensions></Trackpoint><Trackpoint><Time>2008-03-03T23:05:50Z</Time><Position><LatitudeDegrees>35.864151</LatitudeDegrees><LongitudeDegrees>-78.878601</LongitudeDegrees></Position><AltitudeMeters>66.949</AltitudeMeters><DistanceMeters>11361.405</DistanceMeters><Cadence>84</Cadence><Extensions><TPX xmlns=\"http://www.garmin.com/xmlschemas/ActivityExtension/v2\"><Watts>191</Watts></TPX></Extensions></Trackpoint><Trackpoint><Time>2008-03-03T23:05:51Z</Time><Position><LatitudeDegrees>35.864086</LatitudeDegrees><LongitudeDegrees>-78.878684</LongitudeDegrees></Position><AltitudeMeters>66.949</AltitudeMeters><DistanceMeters>11371.760</DistanceMeters><Cadence>84</Cadence><Extensions><TPX xmlns=\"http://www.garmin.com/xmlschemas/ActivityExtension/v2\"><Watts>191</Watts></TPX></Extensions></Trackpoint><Trackpoint><Time>2008-03-03T23:05:52Z</Time><Position><LatitudeDegrees>35.864017</LatitudeDegrees><LongitudeDegrees>-78.878758</LongitudeDegrees></Position><AltitudeMeters>66.949</AltitudeMeters><DistanceMeters>11381.933</DistanceMeters><Cadence>0</Cadence></Trackpoint><Trackpoint><Time>2008-03-03T23:05:53Z</Time><Position><LatitudeDegrees>35.863958</LatitudeDegrees><LongitudeDegrees>-78.878832</LongitudeDegrees></Position><AltitudeMeters>66.468</AltitudeMeters><DistanceMeters>11391.171</DistanceMeters><Cadence>0</Cadence></Trackpoint><Trackpoint><Time>2008-03-03T23:05:54Z</Time><Position><LatitudeDegrees>35.863937</LatitudeDegrees><LongitudeDegrees>-78.878942</LongitudeDegrees></Position><AltitudeMeters>65.507</AltitudeMeters><DistanceMeters>11401.371</DistanceMeters><Cadence>17</Cadence></Trackpoint><Trackpoint><Time>2008-03-03T23:05:55Z</Time><Position><LatitudeDegrees>35.863962</LatitudeDegrees><LongitudeDegrees>-78.879042</LongitudeDegrees></Position><AltitudeMeters>65.026</AltitudeMeters><DistanceMeters>11410.849</DistanceMeters><Cadence>74</Cadence><Extensions><TPX xmlns=\"http://www.garmin.com/xmlschemas/ActivityExtension/v2\"><Watts>416</Watts></TPX></Extensions></Trackpoint><Trackpoint><Time>2008-03-03T23:05:56Z</Time><Position><LatitudeDegrees>35.864024</LatitudeDegrees><LongitudeDegrees>-78.879109</LongitudeDegrees></Position><AltitudeMeters>65.507</AltitudeMeters><DistanceMeters>11420.108</DistanceMeters><Cadence>77</Cadence><Extensions><TPX xmlns=\"http://www.garmin.com/xmlschemas/ActivityExtension/v2\"><Watts>616</Watts></TPX></Extensions></Trackpoint><Trackpoint><Time>2008-03-03T23:05:57Z</Time><Position><LatitudeDegrees>35.864098</LatitudeDegrees><LongitudeDegrees>-78.879162</LongitudeDegrees></Position><AltitudeMeters>65.507</AltitudeMeters><DistanceMeters>11429.607</DistanceMeters><Cadence>77</Cadence><Extensions><TPX xmlns=\"http://www.garmin.com/xmlschemas/ActivityExtension/v2\"><Watts>628</Watts></TPX></Extensions></Trackpoint><Trackpoint><Time>2008-03-03T23:05:58Z</Time><Position><LatitudeDegrees>35.864171</LatitudeDegrees><LongitudeDegrees>-78.879226</LongitudeDegrees></Position><AltitudeMeters>65.507</AltitudeMeters><DistanceMeters>11439.525</DistanceMeters><Cadence>81</Cadence><Extensions><TPX xmlns=\"http://www.garmin.com/xmlschemas/ActivityExtension/v2\"><Watts>655</Watts></TPX></Extensions></Trackpoint><Trackpoint><Time>2008-03-03T23:05:59Z</Time><Position><LatitudeDegrees>35.864244</LatitudeDegrees><LongitudeDegrees>-78.879299</LongitudeDegrees></Position><AltitudeMeters>65.507</AltitudeMeters><DistanceMeters>11449.930</DistanceMeters><Cadence>81</Cadence><Extensions><TPX xmlns=\"http://www.garmin.com/xmlschemas/ActivityExtension/v2\"><Watts>662</Watts></TPX></Extensions></Trackpoint><Trackpoint><Time>2008-03-03T23:06:00Z</Time><Position><LatitudeDegrees>35.864320</LatitudeDegrees><LongitudeDegrees>-78.879379</LongitudeDegrees></Position><AltitudeMeters>65.988</AltitudeMeters><DistanceMeters>11461.130</DistanceMeters><Cadence>93</Cadence><Extensions><TPX xmlns=\"http://www.garmin.com/xmlschemas/ActivityExtension/v2\"><Watts>898</Watts></TPX></Extensions></Trackpoint><Trackpoint><Time>2008-03-03T23:06:01Z</Time><Position><LatitudeDegrees>35.864401</LatitudeDegrees><LongitudeDegrees>-78.879461</LongitudeDegrees></Position><AltitudeMeters>65.988</AltitudeMeters><DistanceMeters>11472.757</DistanceMeters><Cadence>93</Cadence><Extensions><TPX xmlns=\"http://www.garmin.com/xmlschemas/ActivityExtension/v2\"><Watts>896</Watts></TPX></Extensions></Trackpoint><Trackpoint><Time>2008-03-03T23:06:02Z</Time><Position><LatitudeDegrees>35.864484</LatitudeDegrees><LongitudeDegrees>-78.879540</LongitudeDegrees></Position><AltitudeMeters>65.988</AltitudeMeters><DistanceMeters>11484.492</DistanceMeters><Cadence>95</Cadence><Extensions><TPX xmlns=\"http://www.garmin.com/xmlschemas/ActivityExtension/v2\"><Watts>957</Watts></TPX></Extensions></Trackpoint><Trackpoint><Time>2008-03-03T23:06:03Z</Time><Position><LatitudeDegrees>35.864573</LatitudeDegrees><LongitudeDegrees>-78.879612</LongitudeDegrees></Position><AltitudeMeters>66.949</AltitudeMeters><DistanceMeters>11496.220</DistanceMeters><Cadence>95</Cadence><Extensions><TPX xmlns=\"http://www.garmin.com/xmlschemas/ActivityExtension/v2\"><Watts>921</Watts></TPX></Extensions></Trackpoint><Trackpoint><Time>2008-03-03T23:06:04Z</Time><Position><LatitudeDegrees>35.864665</LatitudeDegrees><LongitudeDegrees>-78.879671</LongitudeDegrees></Position><AltitudeMeters>67.430</AltitudeMeters><DistanceMeters>11507.750</DistanceMeters><Cadence>94</Cadence><Extensions><TPX xmlns=\"http://www.garmin.com/xmlschemas/ActivityExtension/v2\"><Watts>831</Watts></TPX></Extensions></Trackpoint><Trackpoint><Time>2008-03-03T23:06:05Z</Time><Position><LatitudeDegrees>35.864761</LatitudeDegrees><LongitudeDegrees>-78.879719</LongitudeDegrees></Position><AltitudeMeters>68.872</AltitudeMeters><DistanceMeters>11519.301</DistanceMeters><Cadence>94</Cadence><Extensions><TPX xmlns=\"http://www.garmin.com/xmlschemas/ActivityExtension/v2\"><Watts>728</Watts></TPX></Extensions></Trackpoint><Trackpoint><Time>2008-03-03T23:06:06Z</Time><Position><LatitudeDegrees>35.864857</LatitudeDegrees><LongitudeDegrees>-78.879755</LongitudeDegrees></Position><AltitudeMeters>69.352</AltitudeMeters><DistanceMeters>11530.362</DistanceMeters><Cadence>86</Cadence><Extensions><TPX xmlns=\"http://www.garmin.com/xmlschemas/ActivityExtension/v2\"><Watts>484</Watts></TPX></Extensions></Trackpoint><Trackpoint><Time>2008-03-03T23:06:07Z</Time><Position><LatitudeDegrees>35.864948</LatitudeDegrees><LongitudeDegrees>-78.879780</LongitudeDegrees></Position><AltitudeMeters>69.352</AltitudeMeters><DistanceMeters>11540.706</DistanceMeters><Cadence>83</Cadence><Extensions><TPX xmlns=\"http://www.garmin.com/xmlschemas/ActivityExtension/v2\"><Watts>323</Watts></TPX></Extensions></Trackpoint><Trackpoint><Time>2008-03-03T23:06:08Z</Time><Position><LatitudeDegrees>35.865035</LatitudeDegrees><LongitudeDegrees>-78.879798</LongitudeDegrees></Position><AltitudeMeters>69.833</AltitudeMeters><DistanceMeters>11550.413</DistanceMeters><Cadence>79</Cadence><Extensions><TPX xmlns=\"http://www.garmin.com/xmlschemas/ActivityExtension/v2\"><Watts>321</Watts></TPX></Extensions></Trackpoint><Trackpoint><Time>2008-03-03T23:06:09Z</Time><Position><LatitudeDegrees>35.865119</LatitudeDegrees><LongitudeDegrees>-78.879812</LongitudeDegrees></Position><AltitudeMeters>70.313</AltitudeMeters><DistanceMeters>11559.796</DistanceMeters><Cadence>79</Cadence><Extensions><TPX xmlns=\"http://www.garmin.com/xmlschemas/ActivityExtension/v2\"><Watts>320</Watts></TPX></Extensions></Trackpoint><Trackpoint><Time>2008-03-03T23:06:10Z</Time><Position><LatitudeDegrees>35.865200</LatitudeDegrees><LongitudeDegrees>-78.879828</LongitudeDegrees></Position><AltitudeMeters>70.794</AltitudeMeters><DistanceMeters>11568.860</DistanceMeters><Cadence>75</Cadence><Extensions><TPX xmlns=\"http://www.garmin.com/xmlschemas/ActivityExtension/v2\"><Watts>365</Watts></TPX></Extensions></Trackpoint><Trackpoint><Time>2008-03-03T23:06:11Z</Time><Position><LatitudeDegrees>35.865277</LatitudeDegrees><LongitudeDegrees>-78.879848</LongitudeDegrees></Position><AltitudeMeters>71.275</AltitudeMeters><DistanceMeters>11577.578</DistanceMeters><Cadence>73</Cadence><Extensions><TPX xmlns=\"http://www.garmin.com/xmlschemas/ActivityExtension/v2\"><Watts>386</Watts></TPX></Extensions></Trackpoint><Trackpoint><Time>2008-03-03T23:06:12Z</Time><Position><LatitudeDegrees>35.865354</LatitudeDegrees><LongitudeDegrees>-78.879867</LongitudeDegrees></Position><AltitudeMeters>71.755</AltitudeMeters><DistanceMeters>11586.277</DistanceMeters><Cadence>72</Cadence><Extensions><TPX xmlns=\"http://www.garmin.com/xmlschemas/ActivityExtension/v2\"><Watts>399</Watts></TPX></Extensions></Trackpoint><Trackpoint><Time>2008-03-03T23:06:13Z</Time><Position><LatitudeDegrees>35.865436</LatitudeDegrees><LongitudeDegrees>-78.879878</LongitudeDegrees></Position><AltitudeMeters>71.755</AltitudeMeters><DistanceMeters>11595.582</DistanceMeters><Cadence>71</Cadence><Extensions><TPX xmlns=\"http://www.garmin.com/xmlschemas/ActivityExtension/v2\"><Watts>399</Watts></TPX></Extensions></Trackpoint><Trackpoint><Time>2008-03-03T23:06:14Z</Time><Position><LatitudeDegrees>35.865516</LatitudeDegrees><LongitudeDegrees>-78.879888</LongitudeDegrees></Position><AltitudeMeters>72.236</AltitudeMeters><DistanceMeters>11604.366</DistanceMeters><Cadence>69</Cadence><Extensions><TPX xmlns=\"http://www.garmin.com/xmlschemas/ActivityExtension/v2\"><Watts>383</Watts></TPX></Extensions></Trackpoint><Trackpoint><Time>2008-03-03T23:06:15Z</Time><Position><LatitudeDegrees>35.865589</LatitudeDegrees><LongitudeDegrees>-78.879903</LongitudeDegrees></Position><AltitudeMeters>73.198</AltitudeMeters><DistanceMeters>11612.526</DistanceMeters><Cadence>68</Cadence><Extensions><TPX xmlns=\"http://www.garmin.com/xmlschemas/ActivityExtension/v2\"><Watts>378</Watts></TPX></Extensions></Trackpoint><Tr
